vi "Remove All CSM Bookmarks.vi"(8 "error in (no error)":errorcluster, 11 "CSM-Helper in":refnum<class "CSM-Helper.lvclass">) -> (0 "error out":errorcluster, 3 "CSM-Helper out":refnum<class "CSM-Helper.lvclass">)   [LabVIEW 2017, in "CSM-Helper.lvclass"]
doc: "### Remove All CSM Bookmarks.vi\n\n-- <b>Controls</b> --\n- <b>CSM-Helper in</b>: CSMHelper input\n\n-- <b>Indicators</b> --\n- <b>CSM-Helper out</b>: CSMHelper output"
uses:
  CSM-Helper.lvclass
  Properties/Read Block Diagram Ref.vi
  Utility/_Support/Diagram.llb/csmHelper-Diagram.lvlib
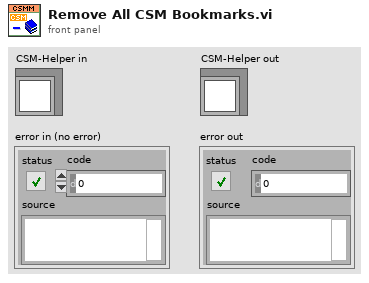
[diagram p1: front panel]
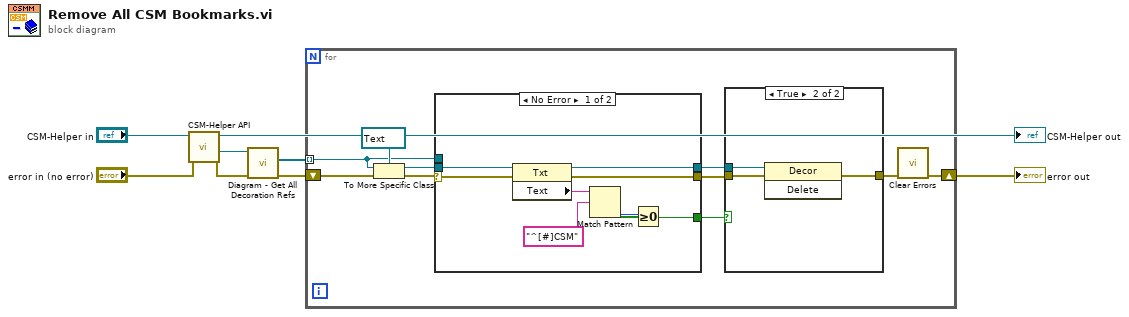
[diagram p0: block diagram]
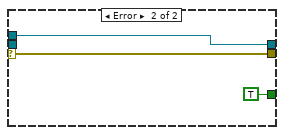
[diagram p2: hidden frame]
diagram:
  n1 = call-poly "CSM-Helper API.vi"("error in (no error)"="error in (no error)", "CSM-Helper in"="CSM-Helper in") -> ("error out"=w3:errorcluster, "Diagram"=w4:refnum<vi>, "CSM-Helper out"=→"CSM-Helper out":refnum<class "CSM-Helper.lvclass">)  [unwired: 7 in]
  n2 = call "Diagram - Get All Decoration Refs.vi"("error in (no error)"=w3, "TopLevelDiagram in"=w4) -> ("error out"=w5:errorcluster, "TextRefs"=w6:refnum<vi>[])  [unwired: 7 in, 1 out]
  n3 = for {
    shift-right: [w16] -> w8
    shift-left: w5 -> [w18]
    tunnel: w6 -> [w9] mode=indexing
    n4 = To More Specific Class(target class=refnum<vi> refnum ("reference"), reference=w9, error in=w18) -> (specific class reference=w13:refnum<vi>, error out=w14:errorcluster)
    n5 = case shown="No Error" w14 {
      selector: w14 -> [w25 w28]
      tunnel: w13 -> [w26 _]
      tunnel: [w21 TRUE] -> w12
      tunnel: [w20 w28] -> w11
      tunnel: [w19 w29] -> w10
      tunnel: w9 -> [_ w29]
      frame No Error {
        n6 = property class="Txt"(reference=w26, error in=w25) -> (reference out=w19:refnum<vi>, error out=w20:errorcluster, "Text"=w24:string)
        n7 = Match Pattern(string=w24, regular expression="^[#]CSM") -> (offset past match=w22:i32)  [unwired: 1 in, 3 out]
        n8 = Greater Or Equal To 0?(x=w22) -> (x >= 0?=w21:bool)
      }
      frame Error {
      }
    }
    n9 = case shown="True" w12 {
      tunnel: [w30 w33] -> w17
      tunnel: w11 -> [w30 w32]
      tunnel: w10 -> [_ w31]
      frame False {
      }
      frame True {
        n10 = invoke class="Decor" method="Delete"(reference=w31, error in=w32) -> (error out=w33:errorcluster)  [unwired: 1 in, 2 out]
      }
    }
    n11 = call <vilib>:"Clear Errors.vi"("error in (no error)"=w17) -> ("error out"=w16:errorcluster)  [unwired: 5 in, 1 out]
  }
  "error out" <- w8
